vi "WireCaseStructureIndicator.vi"(8 "error in (no error)":errorcluster, 10 "Error terminals":T1, 11 "CaseStructure in":refnum<vi>) -> (0 "error out":errorcluster, 2 "Error terminals (dup)":T1, 3 "CaseStructure (dup)":refnum<vi>)   [LabVIEW 2017, in "ErrorStructureDrawer.lvlib"]
doc: "Draws a wire between the case structure's selector terminal (in the \"Error\" case) and either the error indicator (if it was created by this script) or a tunnel in the case structure (if there was already an error indicator)."
uses:
  ErrorStructureDrawer.lvlib
  Controls/ErrorTerminals.ctl
  <vilib>/regexp/Match Regular Expression.xnode
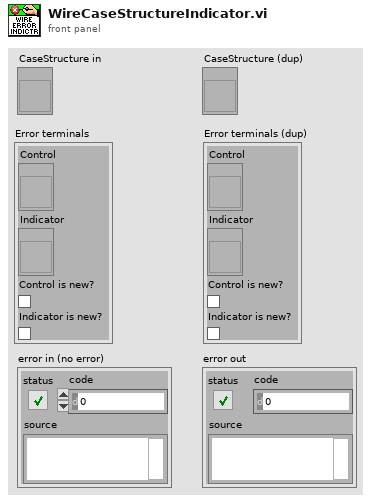
[diagram p1: front panel]
types:
  T1 = typedef "ErrorStructureDrawer.lvlib/ErrorTerminals.ctl" = cluster{"Control":refnum<vi>, "Indicator":refnum<vi>, "Control is new?":bool, "Indicator is new?":bool}
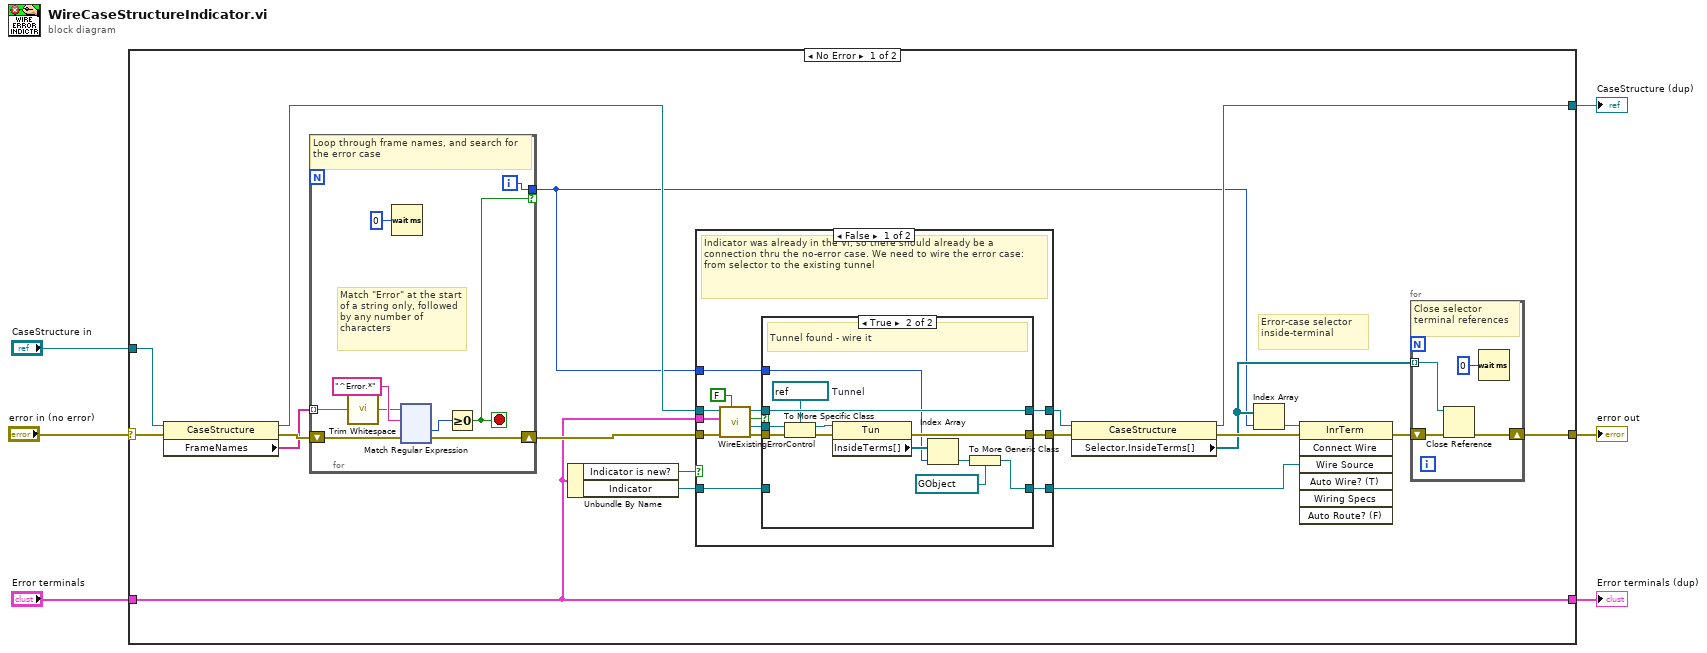
[diagram p0: block diagram]
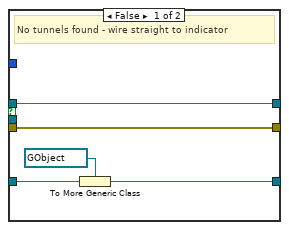
[diagram p2: hidden frame]
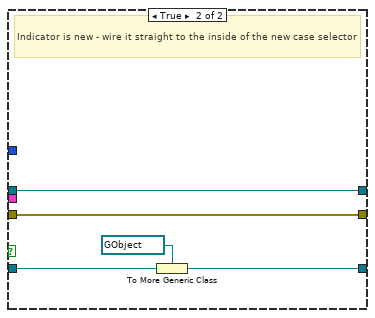
[diagram p3: hidden frame]
diagram:
  n1 = case shown="No Error" "error in (no error)" {
    selector: "error in (no error)" -> [w18 w190]
    tunnel: "Error terminals" -> [w15 w189]
    tunnel: [w10 w188] -> w5
    tunnel: [w25 w190] -> w4
    tunnel: "CaseStructure in" -> [w19 w188]
    tunnel: [w15 w189] -> w2
    frame No Error {
      # "Error-case selector inside-terminal"
      n2 = property class="CaseStructure"(reference=w19, error in=w18) -> (reference out=w14:refnum<vi>, error out=w21:errorcluster, "FrameNames"=w20:string[])
      n3 = for {
        tunnel: w20 -> [w69] mode=indexing
        shift-right: [w65] -> w16
        shift-left: w21 -> [w64]
        tunnel: [w63] -> w7 if=w62
        i -> [w63]
        stop <- w62 stop-if-true
        # "Match \"Error\" at the start of a string only, followed by any number of characters"
        # "Loop through frame names, and search for the error case"
        n4 = call <vilib>:"Trim Whitespace.vi"("string"=w69) -> ("trimmed string"=w66:string)  [unwired: 1 in]
        n5 = Wait (ms)(milliseconds to wait=u32 0) -> ()  [unwired: 1 out]
        n6 = xnode "Match Regular Expression"("input string"=w66, "regular expression"="^Error.*", "error in"=w64) -> ("offset past match"=w67:i32, "error out"=w65:errorcluster)  [unwired: 3 in, 3 out]
        n7 = Greater Or Equal To 0?(x=w67) -> (x >= 0?=w62:bool)
      }
      n8 = Unbundle By Name(w15) -> ("Indicator is new?"=w17:bool, "Indicator"=w22:refnum<vi>)
      n9 = case shown="False" w17 {
        tunnel: [w32 w60] -> w23
        tunnel: w22 -> [w33 w59]
        tunnel: w16 -> [w38 w56]
        tunnel: w15 -> [w37 _]
        tunnel: [w28 w56] -> w13
        tunnel: w14 -> [w36 w57]
        tunnel: [w30 w57] -> w11
        tunnel: w7 -> [w26 _]
        frame False {
          # "Indicator was already in the VI, so there should already be a connection thru the no-error case. We need to wire the error case: from selector to the existing tunnel"
          n10 = call "WireExistingErrorControl.vi"("Control [t] / indicator [f]"=FALSE, "error in (no error)"=w38, "Error terminals"=w37, "CaseStructure in"=w36) -> ("error out"=w29:errorcluster, "Tunnel ref"=w27:refnum<vi>, "Existing wiring used?"=w34:bool, "CaseStructure (dup)"=w31:refnum<vi>)  [unwired: 4 in]
          n11 = case shown="True" w34 {
            tunnel: w33 -> [w42 _]
            tunnel: [w41 w44] -> w32
            tunnel: w31 -> [w40 w55]
            tunnel: [w40 w55] -> w30
            tunnel: w29 -> [w39 w54]
            tunnel: [w39 w49] -> w28
            tunnel: w27 -> [_ w53]
            tunnel: w26 -> [_ w47]
            frame False {
              # "No tunnels found - wire straight to indicator"
              n12 = To More Generic Class(target class=refnum<vi> refnum ("Wire Source"), reference=w42) -> (generic class reference=w41:refnum<vi>)
            }
            frame True {
              w52 = refnum<vi> refnum  # Tunnel
              # "Tunnel found - wire it"
              n13 = To More Specific Class(target class=w52, reference=w53, error in=w54) -> (specific class reference=w51:refnum<vi>, error out=w48:errorcluster)
              n14 = property class="Tun"(reference=w51, error in=w48) -> (error out=w49:errorcluster, "InsideTerms[]"=w50:refnum<vi>[])  [unwired: 1 out]
              n15 = Index Array(array=w50, index=w47) -> (element=w45:refnum<vi>)
              n16 = To More Generic Class(target class=refnum<vi> refnum ("Wire Source"), reference=w45) -> (generic class reference=w44:refnum<vi>)
            }
          }
        }
        frame True {
          # "Indicator is new - wire it straight to the inside of the new case selector"
          n17 = To More Generic Class(target class=refnum<vi> refnum ("Wire Source"), reference=w59) -> (generic class reference=w60:refnum<vi>)
        }
      }
      n18 = property class="CaseStructure"(reference=w11, error in=w13) -> (reference out=w10:refnum<vi>, error out=w12:errorcluster, "Selector.InsideTerms[]"=w8:refnum<vi>[])
      n19 = Index Array(array=w8, index=w7) -> (element=w9:refnum<vi>)
      n20 = invoke class="InrTerm" method="Connect Wire"(reference=w9, error in=w12, "Wire Source"=w23) -> (error out=w24:errorcluster)  [unwired: 4 in, 6 out]
      n21 = for {
        tunnel: w8 -> [w186] mode=indexing
        shift-right: [w185] -> w25
        shift-left: w24 -> [w187]
        # "Close selector terminal references"
        n22 = Close Reference(reference=w186, error in (no error)=w187) -> (error out=w185:errorcluster)
        n23 = Wait (ms)(milliseconds to wait=u32 0) -> ()  [unwired: 1 out]
      }
    }
    frame Error {
    }
  }
  "CaseStructure (dup)" <- w5
  "error out" <- w4
  "Error terminals (dup)" <- w2
